vi "H5Pset_filter.vi"(5 "cd_values":u32[](array[numeric]), 6 "error in (no error)":errorcluster, 7 "Filter Flag":T1 items=["H5Z_FLAG_MANDATORY"=0, "H5Z_FLAG_OPTIONAL"=1, "H5Z_FLAG_REVERSE"=256, "H5Z_FLAG_SKIP_EDC"=512], 8 "Filter":T2 items=["H5Z_FILTER_ERROR"=-1, "H5Z_FILTER_NONE"=0, "H5Z_FILTER_DEFLATE"=1, "H5Z_FILTER_SHUFFLE"=2, "H5Z_FILTER_FLETCHER32"=3, "H5Z_FILTER_SZIP"=4], 9 "HDF5 Property Ref":T3) -> (0 "error out":errorcluster, 3 "HDF5 Ref out":T3)   [LabVIEW 2017]
doc: "Adds a filter to the filter pipeline."
uses:
  <vilib>/UPVI/lvhdf5/library.llb/HDF5 Ref.ctl
  <vilib>/UPVI/lvhdf5/property.llb/H5Z_filter_t.ctl
  <vilib>/UPVI/lvhdf5/property.llb/H5Z_flag_t.ctl
  <vilib>/UPVI/lvhdf5/property.llb/H5D_layout_t.ctl
  <vilib>/UPVI/lvhdf5/hdf5.dll
panel:
  # "LVHDF5 Toolkit\nCopyright (c) 2005-2013 by Jason D. Sommerville\nCopyright (c) 2014 by UPVI, LLC.\n\nThis use and distribution of this file is governed by the terms found in \nLICENSE.txt distributed with this toolkit and installed at\n <user.lib>\\_lvhdf5\\LICENSE.txt"
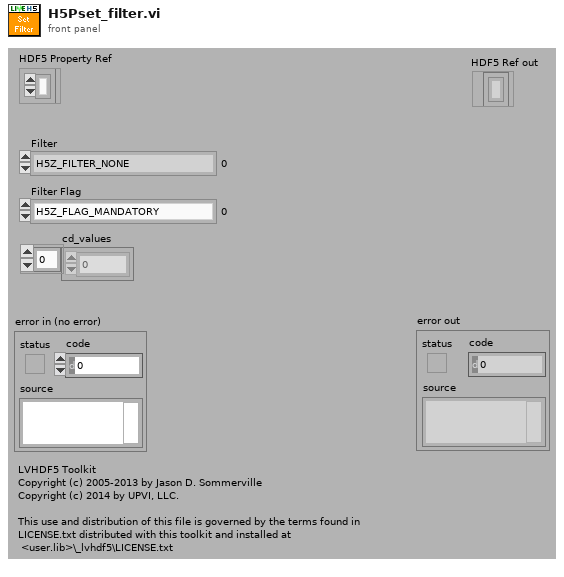
[diagram p1: front panel]
types:
  T1 = typedef "H5Z_flag_t.ctl" = u32
  T2 = typedef "H5Z_filter_t.ctl" = i32
  T3 = typedef "HDF5 Ref.ctl" = refnum<k1>
  T4 = typedef "H5D_layout_t.ctl" = i32
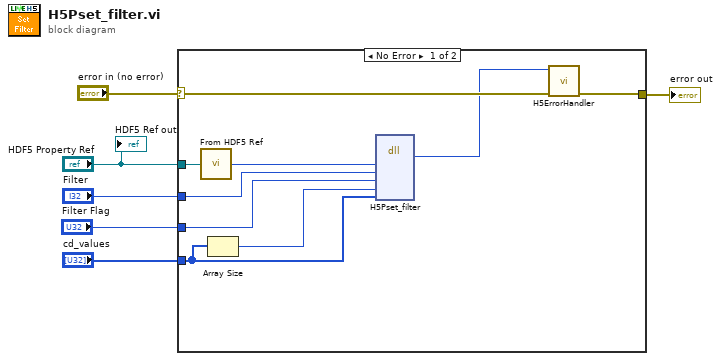
[diagram p0: block diagram]
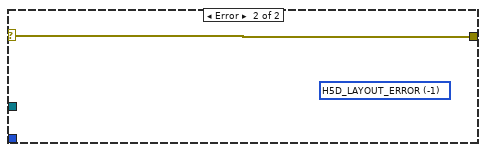
[diagram p2: hidden frame]
diagram:
  n1 = case shown="No Error" "error in (no error)" {
    selector: "error in (no error)" -> [w15 w16]
    tunnel: [w14 w16] -> w5
    tunnel: "HDF5 Property Ref" -> [w13 _]
    tunnel: "Filter" -> [w10 _]
    tunnel: "Filter Flag" -> [w9 _]
    tunnel: "cd_values" -> [w8 _]
    frame No Error {
      n2 = call <vilib>:"From HDF5 Ref.vi"("HDF5 Ref"=w13) -> ("I32"=w12:i32)
      n3 = Array Size(array=w8) -> (size(s)=w7:i32)
      n4 = dll-call lib="C:/Program Files/National Instruments/LabVIEW 2017/vi.lib/UPVI/lvhdf5/hdf5.dll" fn="H5Pset_filter"("plist_id"=w12, "filter"=w10, "flags"=w9, "cd_nelmts"=w7, "cd_values"=w8) -> ("return type"=w11:i32)  [unwired: 8 in, 2 out]
      n5 = call <vilib>:"H5ErrorHandler.vi"("error in (no error)"=w15, "herr_t"=w11) -> ("error out"=w14:errorcluster)  [unwired: 3 in, 4 out]
    }
    frame Error {
      (unwired) T4 -1 items=["H5D_LAYOUT_ERROR"=-1, "H5D_COMPACT"=0, "H5D_CONTIGUOUS"=1, "H5D_CHUNKED"=2] ("Layout")
    }
  }
  "error out" <- w5
  "HDF5 Ref out" <- "HDF5 Property Ref"
